vi "DEMO PNA.vi"(8 "error in (no error)":errorcluster, 11 "N5222A Cfg":T1={"ResourceName"="PNA", "Enable"=TRUE, "Channel"=1, "CalFileName"="CalSet_Peisangtsai_040315_apar_-10dBm", "MeasName"="SxxMeas", "TempDatFile"="APARscratch.csv", "Power, dBm"=-30.0, "NumPoints"=201, "Start Freq, Hz"=5000000000.0, "Stop Freq, Hz"=6000000000.0, "NumAverages"=20, "Sweep Type"=0} {"Sweep Type" items=["Linear Frequency", "Log Frequency", "Power Sweep", "CW Time"]; "Stop Freq, Hz" format="%_3p"; "Start Freq, Hz" format="%_3p"}) -> (0 "error out":errorcluster, 1 ".csv file":string, 2 "Cal Files by name":string[](array[string]))   [LabVIEW 2018, in "N5222A PNA.lvclass"]
uses:
  N5222A PNA.lvclass
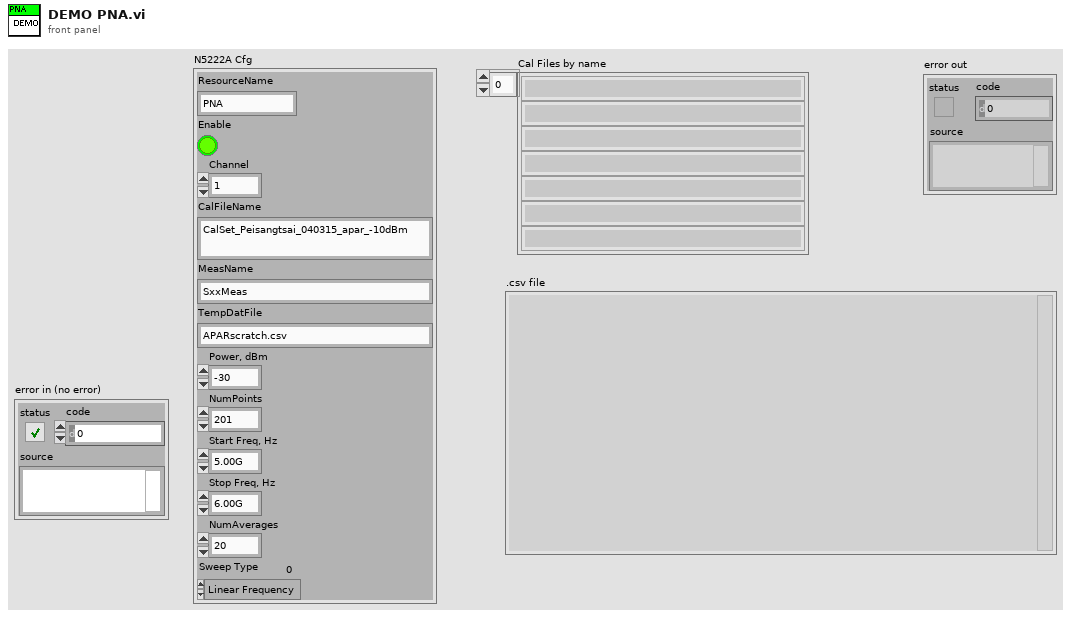
[diagram p1: front panel]
types:
  T1 = cluster{"ResourceName":string, "Enable":bool, "Channel":i32, "CalFileName":string, "MeasName":string, "TempDatFile":string, "Power, dBm":dbl, "NumPoints":i32, "Start Freq, Hz":dbl, "Stop Freq, Hz":dbl, "NumAverages":i32, "Sweep Type":i32}
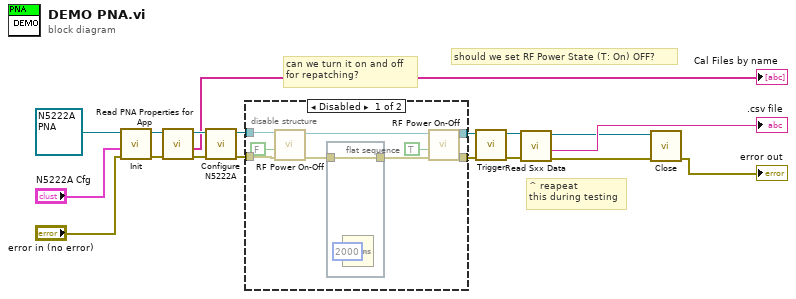
[diagram p0: block diagram]
diagram:
  # "can we turn it on and off\nfor repatching?"
  # "should we set RF Power State (T: On) OFF?"
  # "^ reapeat \nthis during testing"
  n1 = call "Init.vi"("error in (no error)"="error in (no error)", "N5222A Cfg"="N5222A Cfg", "N5222A PNA in"=refnum<class "N5222A PNA.lvclass"> refnum) -> ("error out"=w13:errorcluster, "N5222A PNA out"=w17:refnum<class "N5222A PNA.lvclass">)  [unwired: 7 in]
  n2 = call "Read PNA Properties for App.vi"("error in (no error)"=w13, "N5222A PNA in"=w17) -> ("error out"=w14:errorcluster, "Cal Files by name"=→"Cal Files by name":string[], "N5222A PNA out"=w16:refnum<class "N5222A PNA.lvclass">)  [unwired: 7 in]
  n3 = call "Configure N5222A.vi"("error in (no error)"=w14, "N5222A PNA in"=w16) -> ("error out"=w5:errorcluster, "N5222A PNA out"=w6:refnum<class "N5222A PNA.lvclass">)  [unwired: 8 in]
  n4 = disable-structure shown="Disabled" {
    disable-tunnel: w6 -> [w27 w31]
    disable-tunnel: w5 -> [w26 w30]
    disable-tunnel: [w22 w30] -> w4
    disable-tunnel: [w21 w31] -> w3
    frame Disabled {
      n5 = call "RF Power On-Off.vi"("error in (no error)"=w26, "RF Power State (T: On)"=FALSE, "N5222A PNA in"=w27) -> ("error out"=w24:errorcluster, "N5222A PNA out"=w19:refnum<class "N5222A PNA.lvclass">)  [unwired: 7 in]
      n6 = flat-sequence {
        tunnel: [w28] -> w20
        tunnel: w24 -> [w28]
        frame #0 {
          n7 = Wait (ms)(milliseconds to wait=u32 2000) -> ()  [unwired: 1 out]
        }
      }
      n8 = call "RF Power On-Off.vi"("error in (no error)"=w20, "RF Power State (T: On)"=TRUE, "N5222A PNA in"=w19) -> ("error out"=w22:errorcluster, "N5222A PNA out"=w21:refnum<class "N5222A PNA.lvclass">)  [unwired: 7 in]
    }
    frame Enabled {
    }
  }
  n9 = call "Trigger.vi"("error in (no error)"=w4, "N5222A PNA in"=w3) -> ("error out"=w8:errorcluster, "N5222A PNA out"=w7:refnum<class "N5222A PNA.lvclass">)  [unwired: 8 in]
  n10 = call "Read Sxx Data.vi"("error in (no error)"=w8, "N5222A PNA in"=w7) -> ("error out"=w10:errorcluster, ".csv file"=→".csv file":string, "N5222A PNA out"=w9:refnum<class "N5222A PNA.lvclass">)  [unwired: 7 in]
  n11 = call "Close.vi"("error in (no error)"=w10, "N5222A PNA in"=w9) -> ("error out"=→"error out":errorcluster)  [unwired: 8 in, 1 out]
